vi "Register and Process SAL events.vi"(8 "error in (no error)":errorcluster, 9 "M1M3 Support Events in":refnum<class "M1M3 Support Events.lvclass">, 11 "SAL in":refnum<class "SAL.lvclass">) -> (0 "error out":errorcluster, 3 "SAL out":refnum<class "SAL.lvclass">)   [LabVIEW 2016, in "SAL.lvclass"]
uses:
  SAL.lvclass
  M1M3 Support Events/M1M3 Support Events.lvclass
  Typedefs/SAL Connected.ctl
  M1M3 Support Events/M1M3 Support Events.lvclass/M1M3 Support Events.ctl
  Typedefs/StateTypes.ctl
  SALLV_m1m3/SALLV_m1m3.lvlib
  Typedefs/M1M3SupportEUI_TypeDefs.lvlib
panel:
  out "Boolean":bool
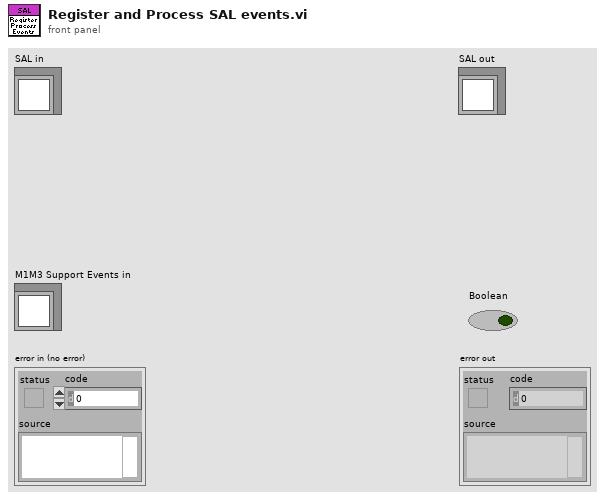
[diagram p1: front panel]
types:
  T1 = typedef "M1M3SupportEUI_TypeDefs.lvlib/SAL Connected.ctl" = cluster{"Is Connected":bool}
  T2 = typedef "M1M3SupportEUI_TypeDefs.lvlib/M1M3 Support Events.ctl" = cluster{"M1M3 Support State":refnum<user-event>, "Inclinometer  Data":refnum<user-event>, "IMS Data":refnum<user-event>, "FA Data":refnum<user-event>, "FA Status":refnum<user-event>, "SAL Connected":refnum<user-event>, "HP Data":refnum<user-event>, "HP Status":refnum<user-event>, "Accelerometer Data":refnum<user-event>, "FPGA Data":refnum<user-event>, "Inclinometer Data":refnum<user-event>}
  T3 = typedef "M1M3SupportEUI_TypeDefs.lvlib/StateTypes.ctl" = u32
  T4 = typedef "SALLV_m1m3.lvlib/logevent_SummaryState.ctl" = cluster{"Timestamp":dbl, "SummaryState":i32, "priority":i32}
  T5 = typedef "SALLV_m1m3.lvlib/IMSData.ctl" = cluster{"Timestamp":dbl, "RawSensorData[8]":dbl[], "XPosition":dbl, "YPosition":dbl, "ZPosition":dbl, "XRotation":dbl, "YRotation":dbl, "ZRotation":dbl}
  T6 = typedef "SALLV_m1m3.lvlib/InclinometerData.ctl" = cluster{"Timestamp":dbl, "InclinometerAngle":dbl}
  T7 = cluster{"Timestamp":dbl, "StaticXSetpoint[156]":dbl[], "StaticYSetpoint[156]":dbl[], "StaticZSetpoint[156]":dbl[], "ElevationXSetpoint[156]":dbl[], "ElevationYSetpoint[156]":dbl[], "ElevationZSetpoint[156]":dbl[], "AzimuthXSetpoint[156]":dbl[], "AzimuthYSetpoint[156]":dbl[], "AzimuthZSetpoint[156]":dbl[], "TemperatureXSetpoint[156]":dbl[], "TemperatureYSetpoint[156]":dbl[], "TemperatureZSetpoint[156]":dbl[], "ActiveOpticsZSetpoint[156]":dbl[], "AberrationZSetpoint[156]":dbl[], "HardpointOffloadXSetpoint[156]":dbl[], "HardpointOffloadYSetpoint[156]":dbl[], "HardpointOffloadZSetpoint[156]":dbl[], "DynamicXSetpoint[156]":dbl[], "DynamicYSetpoint[156]":dbl[], "DynamicZSetpoint[156]":dbl[], "OffsetXSetpoint[156]":dbl[], "OffsetYSetpoint[156]":dbl[], "OffsetZSetpoint[156]":dbl[], "ElevationSetpointPercentage":dbl, "XSetpoint[156]":dbl[], "YSetpoint[156]":dbl[], "ZSetpoint[156]":dbl[], "PrimaryCylinderSetpointCommanded[156]":i32[], "SecondaryCylinderSetpointCommanded[156]":i32[], "BroadcastCounter[156]":u8[], "SlewFlagCommanded[156]":bool[], "PrimaryCylinderForce[156]":sgl[], "SecondaryCylinderForce[156]":sgl[], "ILCFault[156]":bool[], "DCAFault[156]":bool[], "XForce[156]":dbl[], "YForce[156]":dbl[], "ZForce[156]":dbl[]}
  T8 = typedef "SALLV_m1m3.lvlib/ForceActuatorStatus.ctl" = cluster{"Timestamp":dbl, "Mode[156]":u8[], "MajorFault[156]":bool[], "MinorFault[156]":bool[], "FaultOverridden[156]":bool[], "DCAFault[156]":bool[], "WatchdogReset[156]":bool[], "BrownoutDetected[156]":bool[], "EventTrapReset[156]":bool[], "MotorPowerFault[156]":bool[], "SSRPowerFault[156]":bool[], "AUXPowerFault[156]":bool[], "SMCPowerFault[156]":bool[], "DCAOutputsEnabled[156]":bool[], "DCAPowerFault[156]":bool[], "DCAAmplifierAFault[156]":bool[], "DCAAmplifierBFault[156]":bool[], "DCAEventTrapReset[156]":bool[]}
  T9 = typedef "SALLV_m1m3.lvlib/HardpointData.ctl" = cluster{"Timestamp":dbl, "StepsQueued[6]":i32[], "StepsCommanded[6]":i16[], "Force[6]":sgl[], "Encoder[6]":i32[], "ILCFault[6]":bool[], "CWLimitOperated[6]":bool[], "CCWLimitOperated[6]":bool[], "BroadcastCounter[6]":u8[], "Displacement[6]":dbl[], "BreakawayLVDT[6]":sgl[], "DisplacementLVDT[6]":sgl[], "BreakawayPressure[6]":sgl[], "XPosition":dbl, "YPosition":dbl, "ZPosition":dbl, "XRotation":dbl, "YRotation":dbl, "ZRotation":dbl}
  T10 = typedef "SALLV_m1m3.lvlib/HardpointStatus.ctl" = cluster{"Timestamp":dbl, "Mode[6]":u8[], "MajorFault[6]":bool[], "MinorFault[6]":bool[], "FaultOverridden[6]":bool[], "WatchdogReset[6]":bool[], "BrownoutDetected[6]":bool[], "EventTrapReset[6]":bool[], "MotorPowerFault[6]":bool[], "SSRPowerFault[6]":bool[], "AUXPowerFault[6]":bool[], "SMCPowerFault[6]":bool[]}
  T11 = typedef "SALLV_m1m3.lvlib/FPGAData.ctl" = cluster{"Timestamp":dbl, "ModbusTxInternalFIFOOverflow[5]":bool[], "ModbusInvalidInstruction[5]":bool[], "ModbusWaitForRxFrameTimeout[5]":bool[], "ModbusStartBitError[5]":bool[], "ModbusStopBitError[5]":bool[], "ModbusRxDataFIFOOverflow[5]":bool[], "ModbusTxByteCount[5]":u32[], "ModbusTxFrameCount[5]":u32[], "ModbusRxByteCount[5]":u32[], "ModbusRxFrameCount[5]":u32[], "FPGATime":dbl}
  T12 = typedef "SALLV_m1m3.lvlib/AccelerometerData.ctl" = cluster{"Timestamp":dbl, "RawAccelerometerX[2]":dbl[], "RawAccelerometerY[2]":dbl[], "RawAccelerometerZ[4]":dbl[], "AngularAccelerationX":dbl, "AngularAccelerationY":dbl, "AngularAccelerationZ":dbl}
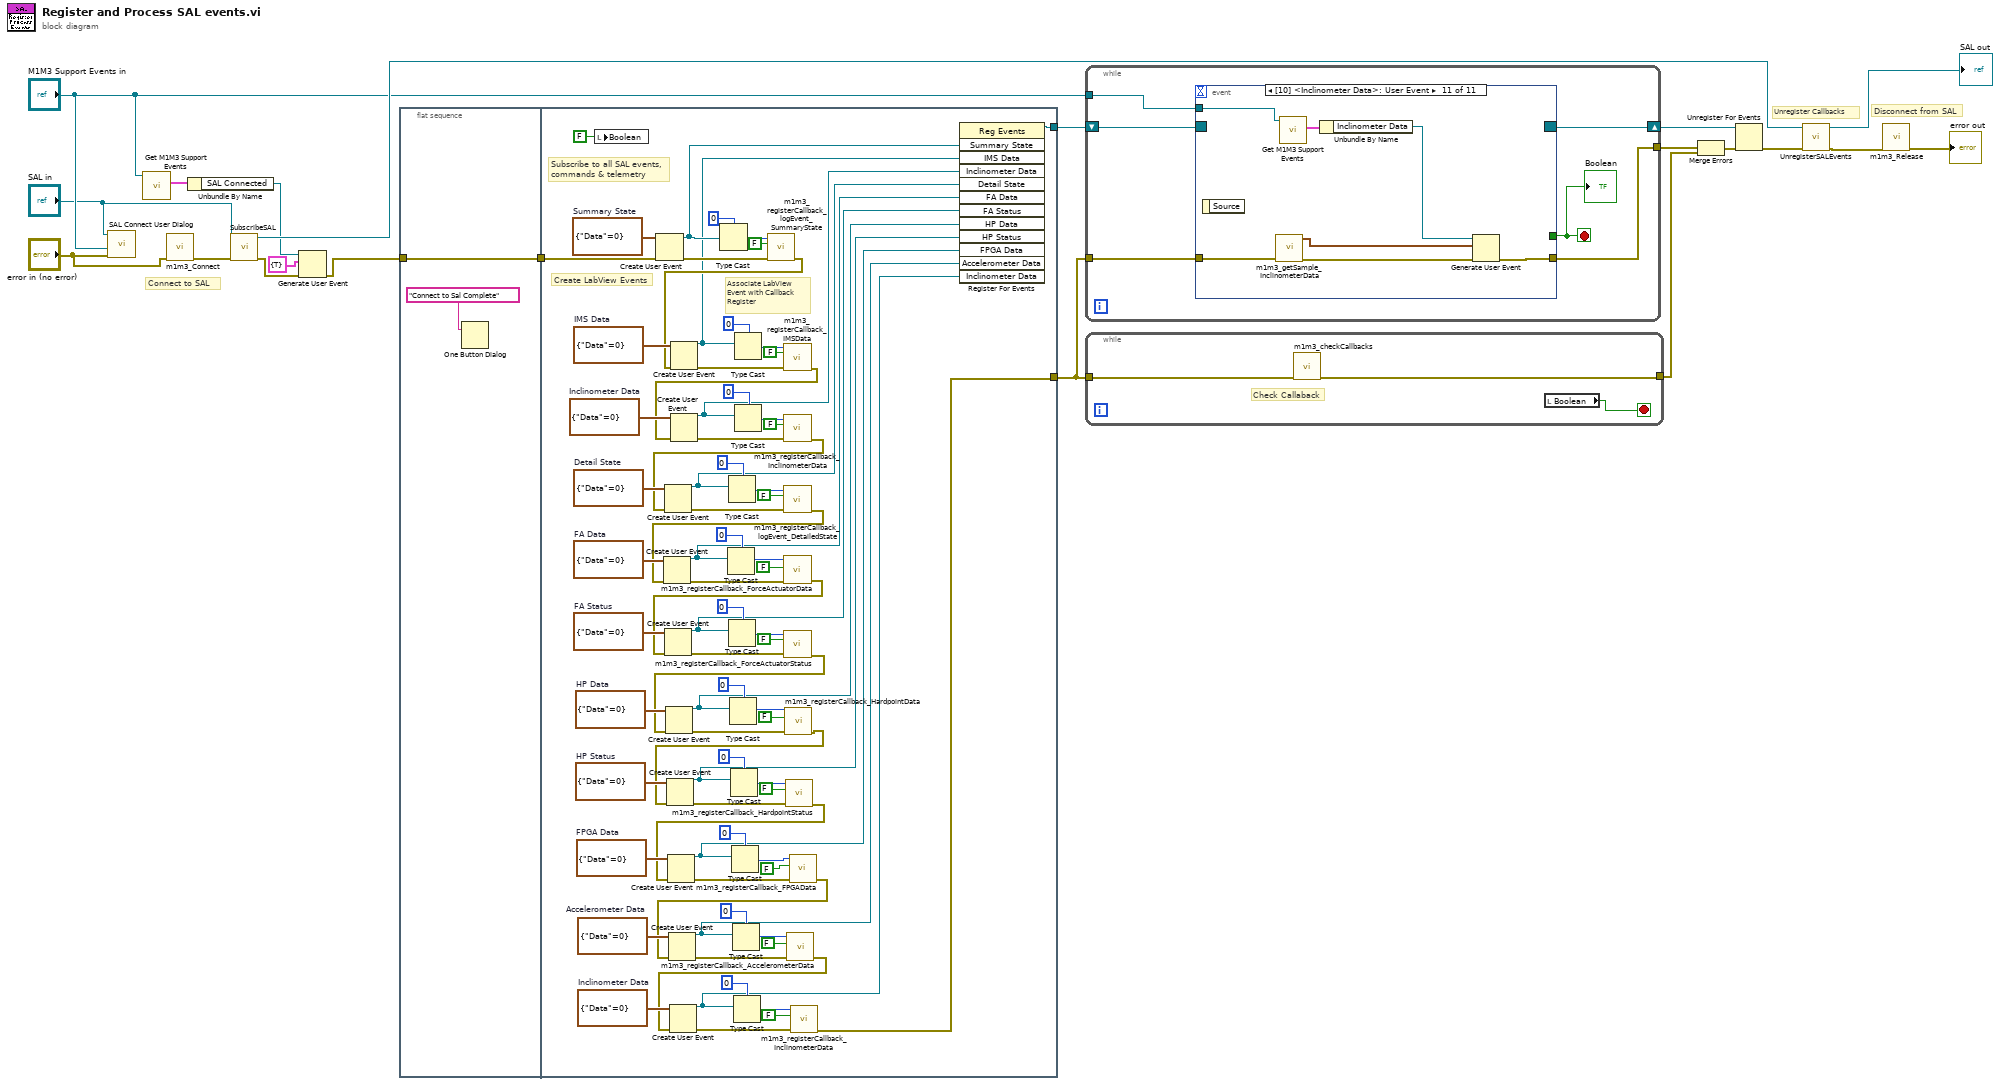
[diagram p0: block diagram]
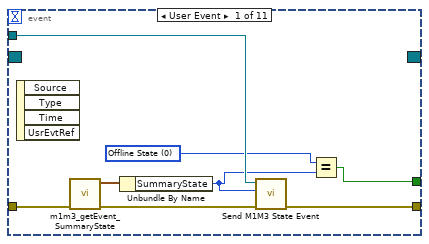
[diagram p2: hidden frame]
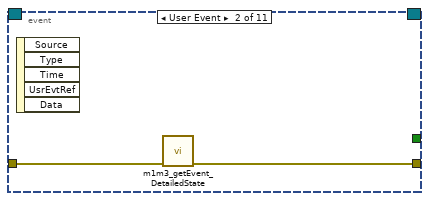
[diagram p3: hidden frame]
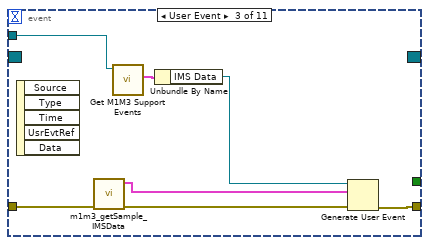
[diagram p4: hidden frame]
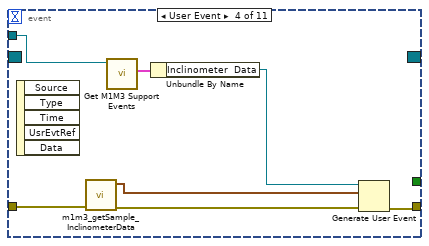
[diagram p5: hidden frame]
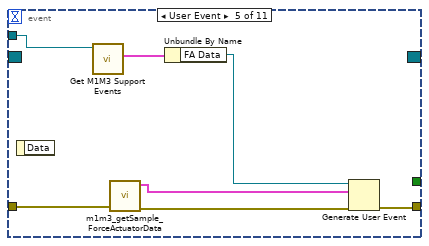
[diagram p6: hidden frame]
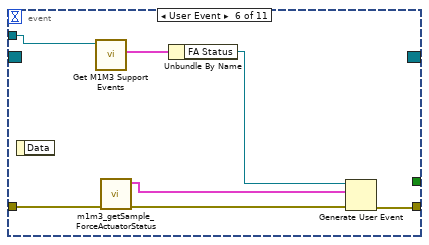
[diagram p7: hidden frame]
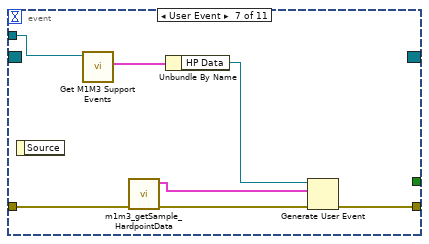
[diagram p8: hidden frame]
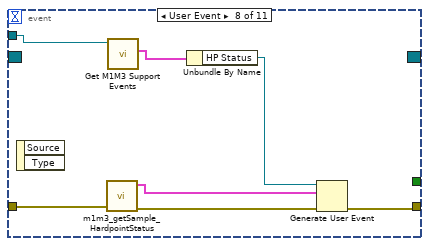
[diagram p9: hidden frame]
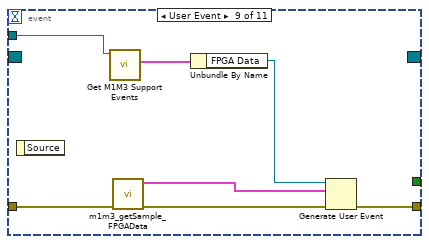
[diagram p10: hidden frame]
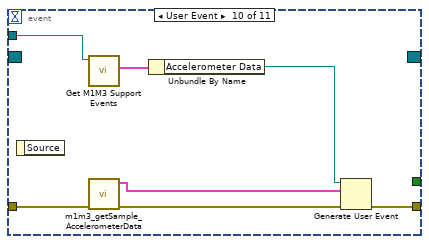
[diagram p11: hidden frame]
diagram:
  # "Disconnect from SAL"
  # "Unregister Callbacks"
  # "Connect to SAL"
  n1 = call "SAL Connect User Dialog.vi"("error in (no error)"="error in (no error)", "M1M3 Support Events in"="M1M3 Support Events in", "SAL in"="SAL in") -> ()  [unwired: 7 in, 2 out]
  n2 = call "Get M1M3 Support Events.vi"("M1M3 Support Events in"="M1M3 Support Events in") -> ("M1M3 Support Events"=w7:T2)  [unwired: 9 in, 1 out]
  n3 = call "m1m3_Connect.vi"("error in (no error)"="error in (no error)") -> ("error out"=w18:errorcluster)  [unwired: 9 in, 1 out]
  n4 = Unbundle By Name(w7) -> ("SAL Connected"=w4:refnum<user-event>)
  n5 = call "SubscribeSAL.vi"("error in (no error)"=w18, "SAL in"="SAL in") -> ("error out"=w6:errorcluster, "SAL out"=w10:refnum<class "SAL.lvclass">)  [unwired: 8 in]
  n6 = Generate User Event(user event=w4, event data cluster=T1 {"Is Connected"=TRUE} ("SAL Connected"), error in=w6) -> (error out=w5:errorcluster)  [unwired: 1 in, 1 out]
  n7 = flat-sequence {
    tunnel: w5 -> [w23]
    tunnel: [w23] -> w9
    tunnel: w9 -> [w101]
    tunnel: [w103] -> w20
    tunnel: [w29] -> w11
    frame #0 {
      n8 = One Button Dialog(message="Connect to Sal Complete") -> ()  [unwired: 1 in, 1 out]
    }
    frame #1 {
      w42 = cluster{"Data":i32} {"Data"=0}  # Inclinometer Data
      w45 = cluster{"Data":i32} {"Data"=0}  # Accelerometer Data
      w41 = cluster{"Data":i32} {"Data"=0}  # FPGA Data
      w59 = cluster{"Data":i32} {"Data"=0}  # HP Status
      w56 = cluster{"Data":i32} {"Data"=0}  # HP Data
      w70 = cluster{"Data":i32} {"Data"=0}  # FA Status
      w73 = cluster{"Data":i32} {"Data"=0}  # FA Data
      w79 = cluster{"Data":i32} {"Data"=0}  # Detail State
      w88 = cluster{"Data":i32} {"Data"=0}  # Inclinometer Data
      w94 = cluster{"Data":i32} {"Data"=0}  # IMS Data
      w102 = cluster{"Data":i32} {"Data"=0}  # Summary State
      # "Associate LabView\nEvent with Callback\nRegister"
      # "Create LabView Events"
      # "Subscribe to all SAL events, \ncommands & telemetry"
      n9 = local write "Boolean"(FALSE ("Boolean")) -> ()
      n10 = Create User Event(user event datatype=w102, error in=w101) -> (user event=w100:refnum<user-event>, error out=w97:errorcluster)
      n11 = Type Cast(type=0, x=w100) -> (*(type *) &x=w98:i32)
      n12 = call "m1m3_registerCallback_logEvent_SummaryState.vi"("error in (no error)"=w97, "skipOld"=FALSE, "handle"=w98) -> ("error out"=w93:errorcluster)  [unwired: 7 in, 1 out]
      n13 = Create User Event(user event datatype=w94, error in=w93) -> (user event=w92:refnum<user-event>, error out=w89:errorcluster)
      n14 = Type Cast(type=0, x=w92) -> (*(type *) &x=w90:i32)
      n15 = call "m1m3_registerCallback_IMSData.vi"("error in (no error)"=w89, "skipOld"=FALSE, "handle"=w90) -> ("error out"=w86:errorcluster)  [unwired: 7 in, 1 out]
      n16 = Create User Event(user event datatype=w88, error in=w86) -> (user event=w82:refnum<user-event>, error out=w85:errorcluster)
      n17 = Type Cast(type=0, x=w82) -> (*(type *) &x=w84:i32)
      n18 = call "m1m3_registerCallback_InclinometerData.vi"("error in (no error)"=w85, "skipOld"=FALSE, "handle"=w84) -> ("error out"=w78:errorcluster)  [unwired: 7 in, 1 out]
      n19 = Create User Event(user event datatype=w79, error in=w78) -> (user event=w77:refnum<user-event>, error out=w76:errorcluster)
      n20 = Type Cast(type=0, x=w77) -> (*(type *) &x=w74:i32)
      n21 = call "m1m3_registerCallback_logEvent_DetailedState.vi"("error in (no error)"=w76, "skipOld"=FALSE, "handle"=w74) -> ("error out"=w69:errorcluster)  [unwired: 7 in, 1 out]
      n22 = Create User Event(user event datatype=w73, error in=w69) -> (user event=w68:refnum<user-event>, error out=w65:errorcluster)
      n23 = Type Cast(type=0, x=w68) -> (*(type *) &x=w67:i32)
      n24 = call "m1m3_registerCallback_ForceActuatorData.vi"("error in (no error)"=w65, "skipOld"=FALSE, "handle"=w67) -> ("error out"=w64:errorcluster)  [unwired: 7 in, 1 out]
      n25 = Create User Event(user event datatype=w70, error in=w64) -> (user event=w63:refnum<user-event>, error out=w60:errorcluster)
      n26 = Type Cast(type=0, x=w63) -> (*(type *) &x=w62:i32)
      n27 = call "m1m3_registerCallback_ForceActuatorStatus.vi"("error in (no error)"=w60, "skipOld"=FALSE, "handle"=w62) -> ("error out"=w55:errorcluster)  [unwired: 7 in, 1 out]
      n28 = Create User Event(user event datatype=w56, error in=w55) -> (user event=w54:refnum<user-event>, error out=w50:errorcluster)
      n29 = Type Cast(type=0, x=w54) -> (*(type *) &x=w51:i32)
      n30 = call "m1m3_registerCallback_HardpointData.vi"("error in (no error)"=w50, "skipOld"=FALSE, "handle"=w51) -> ("error out"=w49:errorcluster)  [unwired: 7 in, 1 out]
      n31 = Create User Event(user event datatype=w59, error in=w49) -> (user event=w53:refnum<user-event>, error out=w46:errorcluster)
      n32 = Type Cast(type=0, x=w53) -> (*(type *) &x=w48:i32)
      n33 = call "m1m3_registerCallback_HardpointStatus.vi"("error in (no error)"=w46, "skipOld"=FALSE, "handle"=w48) -> ("error out"=w39:errorcluster)  [unwired: 7 in, 1 out]
      n34 = Create User Event(user event datatype=w41, error in=w39) -> (user event=w35:refnum<user-event>, error out=w37:errorcluster)
      n35 = Type Cast(type=0, x=w35) -> (*(type *) &x=w38:i32)
      n36 = call "m1m3_registerCallback_FPGAData.vi"("error in (no error)"=w37, "skipOld"=FALSE, "handle"=w38) -> ("error out"=w36:errorcluster)  [unwired: 7 in, 1 out]
      n37 = Create User Event(user event datatype=w45, error in=w36) -> (user event=w34:refnum<user-event>, error out=w26:errorcluster)
      n38 = Type Cast(type=0, x=w34) -> (*(type *) &x=w28:i32)
      n39 = call "m1m3_registerCallback_AccelerometerData.vi"("error in (no error)"=w26, "skipOld"=FALSE, "handle"=w28) -> ("error out"=w25:errorcluster)  [unwired: 7 in, 1 out]
      n40 = Create User Event(user event datatype=w42, error in=w25) -> (user event=w33:refnum<user-event>, error out=w30:errorcluster)
      n41 = Type Cast(type=0, x=w33) -> (*(type *) &x=w32:i32)
      n42 = call "m1m3_registerCallback_InclinometerData.vi"("error in (no error)"=w30, "skipOld"=FALSE, "handle"=w32) -> ("error out"=w29:errorcluster)  [unwired: 7 in, 1 out]
      n43 = register-events(w100, w92, w82, w77, w68, w63, w54, w53, w35, w34, w33) -> (reference out=w103:refnum<event-registration>)  [unwired: 2 in, 1 out]
    }
  }
  n44 = while {
    shift-right: [w108] -> w19
    shift-left: w20 -> [w109]
    tunnel: w11 -> [w107]
    tunnel: "M1M3 Support Events in" -> [w106]
    tunnel: [w105] -> w16
    stop <- w104 stop-if-true
    n45 = event shown="[10] <Inclinometer Data>: User Event" {
      selector: w109 -> [_ _ _ _ _ _ _ _ _ _ _]
      dyn-events: [_ _ _ _ _ _ _ _ _ _ _] -> w108
      timeout: _ -> [_ _ _ _ _ _ _ _ _ _ _]
      tunnel: w107 -> [w117 w119 w126 w133 w140 w147 w151 w160 w167 w173 w181]
      tunnel: w106 -> [w116 _ w124 w131 w139 w146 w154 w161 w168 w175 w182]
      tunnel: [w113 w118 w122 w129 w135 w144 w152 w155 w166 w174 w179] -> w105
      tunnel: [w110 _ _ _ _ _ _ _ _ _ _] -> w104
      event User Event {
        w112 = T3 0 items=["Offline State"=0, "Fault State"=4294967295, "Standby State"=16777216, "Disabled State"=33554432, "Enabled State"=50331648, "Parked State"=50331649, "Raising State"=50331650, "Active State"=50331651, "Lowering State"=50331652, "Engineering State"=50397184, "Parked Engineering State"=50397185, "Raising Engineering State"=50397186, "Active Engineering State"=50397187, "Lowering Engineering State"=50397188] ("y")
        n46 = event-data() -> ()  [unwired: 1 in, 4 out]
        n47 = call "m1m3_getEvent_SummaryState.vi"("error in (no error)"=w117) -> ("error out"=w114:errorcluster, "logevent_SummaryState_Ctl out"=w115:T4)  [unwired: 8 in, 1 out]
        n48 = Unbundle By Name(w115) -> ("SummaryState"=w111:i32)
        n49 = call "Send M1M3 State Event.vi"("error in (no error)"=w114, "M1M3 Support State"=w111, "M1M3 Support Events in"=w116) -> ("error out"=w113:errorcluster)  [unwired: 7 in, 1 out]
        n50 = Equal?(x=w112, y=w111) -> (x = y?=w110:bool)
      }
      event User Event {
        n51 = event-data() -> ()  [unwired: 1 in, 5 out]
        n52 = call "m1m3_getEvent_DetailedState.vi"("error in (no error)"=w119) -> ("error out"=w118:errorcluster)  [unwired: 8 in, 2 out]
      }
      event User Event {
        n53 = event-data() -> ()  [unwired: 1 in, 5 out]
        n54 = call "m1m3_getSample_IMSData.vi"("error in (no error)"=w126) -> ("error out"=w123:errorcluster, "IMSData_Ctl out"=w121:T5)  [unwired: 8 in, 1 out]
        n55 = call "Get M1M3 Support Events.vi"("M1M3 Support Events in"=w124) -> ("M1M3 Support Events"=w125:T2)  [unwired: 9 in, 1 out]
        n56 = Unbundle By Name(w125) -> ("IMS Data"=w120:refnum<user-event>)
        n57 = Generate User Event(user event=w120, event data cluster=w121, error in=w123) -> (error out=w122:errorcluster)  [unwired: 1 in, 1 out]
      }
      event User Event {
        n58 = event-data() -> ()  [unwired: 1 in, 5 out]
        n59 = call "m1m3_getSample_InclinometerData.vi"("error in (no error)"=w133) -> ("error out"=w130:errorcluster, "InclinometerData_Ctl out"=w128:T6)  [unwired: 8 in, 1 out]
        n60 = call "Get M1M3 Support Events.vi"("M1M3 Support Events in"=w131) -> ("M1M3 Support Events"=w132:T2)  [unwired: 9 in, 1 out]
        n61 = Unbundle By Name(w132) -> ("Inclinometer  Data"=w127:refnum<user-event>)
        n62 = Generate User Event(user event=w127, event data cluster=w128, error in=w130) -> (error out=w129:errorcluster)  [unwired: 1 in, 1 out]
      }
      event User Event {
        n63 = event-data() -> ()  [unwired: 1 in, 1 out]
        n64 = call "Get M1M3 Support Events.vi"("M1M3 Support Events in"=w139) -> ("M1M3 Support Events"=w138:T2)  [unwired: 9 in, 1 out]
        n65 = call "m1m3_getSample_ForceActuatorData.vi"("error in (no error)"=w140) -> ("error out"=w137:errorcluster, "ForceActuatorData_Ctl out"=w134:T7)  [unwired: 8 in, 1 out]
        n66 = Unbundle By Name(w138) -> ("FA Data"=w136:refnum<user-event>)
        n67 = Generate User Event(user event=w136, event data cluster=w134, error in=w137) -> (error out=w135:errorcluster)  [unwired: 1 in, 1 out]
      }
      event User Event {
        n68 = event-data() -> ()  [unwired: 1 in, 1 out]
        n69 = call "Get M1M3 Support Events.vi"("M1M3 Support Events in"=w146) -> ("M1M3 Support Events"=w145:T2)  [unwired: 9 in, 1 out]
        n70 = call "m1m3_getSample_ForceActuatorStatus.vi"("error in (no error)"=w147) -> ("error out"=w142:errorcluster, "ForceActuatorStatus_Ctl out"=w141:T8)  [unwired: 8 in, 1 out]
        n71 = Unbundle By Name(w145) -> ("FA Status"=w143:refnum<user-event>)
        n72 = Generate User Event(user event=w143, event data cluster=w141, error in=w142) -> (error out=w144:errorcluster)  [unwired: 1 in, 1 out]
      }
      event User Event {
        n73 = event-data() -> ()  [unwired: 1 in, 1 out]
        n74 = call "Get M1M3 Support Events.vi"("M1M3 Support Events in"=w154) -> ("M1M3 Support Events"=w153:T2)  [unwired: 9 in, 1 out]
        n75 = call "m1m3_getSample_HardpointData.vi"("error in (no error)"=w151) -> ("error out"=w150:errorcluster, "HardpointData_Ctl out"=w149:T9)  [unwired: 8 in, 1 out]
        n76 = Unbundle By Name(w153) -> ("HP Data"=w148:refnum<user-event>)
        n77 = Generate User Event(user event=w148, event data cluster=w149, error in=w150) -> (error out=w152:errorcluster)  [unwired: 1 in, 1 out]
      }
      event User Event {
        n78 = event-data() -> ()  [unwired: 1 in, 2 out]
        n79 = call "m1m3_getSample_HardpointStatus.vi"("error in (no error)"=w160) -> ("error out"=w159:errorcluster, "HardpointStatus_Ctl out"=w158:T10)  [unwired: 8 in, 1 out]
        n80 = call "Get M1M3 Support Events.vi"("M1M3 Support Events in"=w161) -> ("M1M3 Support Events"=w157:T2)  [unwired: 9 in, 1 out]
        n81 = Unbundle By Name(w157) -> ("HP Status"=w156:refnum<user-event>)
        n82 = Generate User Event(user event=w156, event data cluster=w158, error in=w159) -> (error out=w155:errorcluster)  [unwired: 1 in, 1 out]
      }
      event User Event {
        n83 = event-data() -> ()  [unwired: 1 in, 1 out]
        n84 = call "Get M1M3 Support Events.vi"("M1M3 Support Events in"=w168) -> ("M1M3 Support Events"=w164:T2)  [unwired: 9 in, 1 out]
        n85 = call "m1m3_getSample_FPGAData.vi"("error in (no error)"=w167) -> ("error out"=w165:errorcluster, "FPGAData_Ctl out"=w162:T11)  [unwired: 8 in, 1 out]
        n86 = Unbundle By Name(w164) -> ("FPGA Data"=w163:refnum<user-event>)
        n87 = Generate User Event(user event=w163, event data cluster=w162, error in=w165) -> (error out=w166:errorcluster)  [unwired: 1 in, 1 out]
      }
      event User Event {
        n88 = event-data() -> ()  [unwired: 1 in, 1 out]
        n89 = call "Get M1M3 Support Events.vi"("M1M3 Support Events in"=w175) -> ("M1M3 Support Events"=w171:T2)  [unwired: 9 in, 1 out]
        n90 = call "m1m3_getSample_AccelerometerData.vi"("error in (no error)"=w173) -> ("error out"=w172:errorcluster, "AccelerometerData_Ctl out"=w169:T12)  [unwired: 8 in, 1 out]
        n91 = Unbundle By Name(w171) -> ("Accelerometer Data"=w170:refnum<user-event>)
        n92 = Generate User Event(user event=w170, event data cluster=w169, error in=w172) -> (error out=w174:errorcluster)  [unwired: 1 in, 1 out]
      }
      event User Event {
        n93 = event-data() -> ()  [unwired: 1 in, 1 out]
        n94 = call "m1m3_getSample_InclinometerData.vi"("error in (no error)"=w181) -> ("error out"=w180:errorcluster, "InclinometerData_Ctl out"=w176:T6)  [unwired: 8 in, 1 out]
        n95 = call "Get M1M3 Support Events.vi"("M1M3 Support Events in"=w182) -> ("M1M3 Support Events"=w178:T2)  [unwired: 9 in, 1 out]
        n96 = Unbundle By Name(w178) -> ("Inclinometer Data"=w177:refnum<user-event>)
        n97 = Generate User Event(user event=w177, event data cluster=w176, error in=w180) -> (error out=w179:errorcluster)  [unwired: 1 in, 1 out]
      }
    }
    "Boolean" <- w104
  }
  n98 = while {
    tunnel: w11 -> [w184]
    tunnel: [w183] -> w15
    stop <- w185 stop-if-true
    # "Check Callaback"
    n99 = call "m1m3_checkCallbacks.vi"("error in (no error)"=w184) -> ("error out"=w183:errorcluster)  [unwired: 10 in]
    n100 = local read "Boolean"() -> (w185:bool)
  }
  n101 = Merge Errors(w16, w15) -> (w17:errorcluster)
  n102 = Unregister For Events(event registration refnum=w19, error in=w17) -> (error out=w14:errorcluster)
  n103 = call "UnregisterSALEvents.vi"("error in (no error)"=w14, "SAL in"=w10) -> ("error out"=w13:errorcluster, "SAL out"=→"SAL out":refnum<class "SAL.lvclass">)  [unwired: 8 in]
  n104 = call "m1m3_Release.vi"("error in (no error)"=w13) -> ("error out"=→"error out":errorcluster)  [unwired: 9 in, 1 out]
